vi "Homescreen.vi"() -> ()   [LabVIEW 2015]
uses:
  Home tab state.ctl
  Home state.ctl
  Undelivered instance.ctl
  <vilib>/Utility/sysdir.llb/System Directory Type.ctl
  <vilib>/Utility/config.llb/NI_LVConfig.lvlib
panel:
  out "Tab Control":T1
  in  "Month Cancel":bool
  in  "Month next":bool
  in  "Month reset":bool
  in  "Year":i32=1900
  in  "Month":i32(ring) items=["January", "February", "March", "April", "May", "June", "July", "August", "September", "October", "November", "December"]
  in  "Undelivered instances":i32(listbox)
  out "Total cost":dbl
  in  "Undelivered cancel":bool
  in  "Undelivered Back":bool
  in  "Undelivered next":bool
  in  "Undelivered clear":bool
  in  "Undelivered add":bool
  in  "Undelivered remove":bool
  in  "Save back":bool
  in  "Save exit":bool
  out "Successfully copied":string caption="Config Message"
  in  "Breakdown copy":bool
  out "Breakdown by newspaper":string
  # "This app calculates the total cost of your newspapers for a given month. Please select the month and year you would like to calculate for and then click Next. You will then\nbe able to enter the details of any instances where newspaper(s) were not delivered."
  # "Please enter the details of instances of missing deliveries (if any) and then click Next. You will then be able to copy the break-down and save the data.\n\nClick Add instance to add an instance, and Remove instance to delete the selected instance."
  # "The box below shows you the costs broken down by newspaper. Click Copy to clipboard and save to records to save this to the logs, and copy it to the clipboard.\n\nClick Exit to finish and close the application."
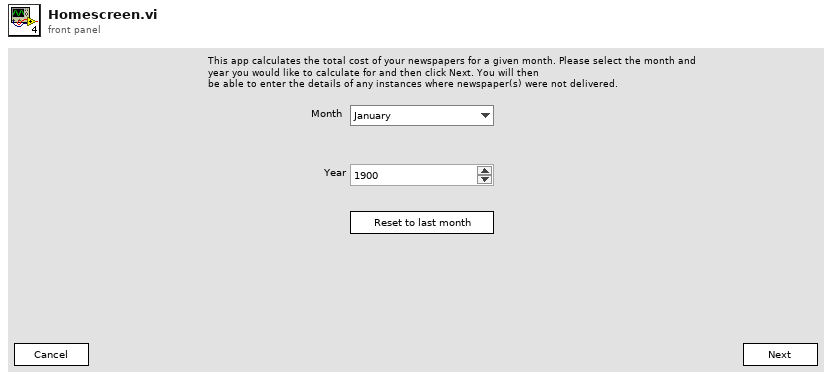
[diagram p1: front panel]
types:
  T1 = typedef "Home tab state.ctl" = enum32{"Pick month", "Select undelivered", "Copy and save"}
  T2 = typedef "Undelivered instance.ctl" = cluster{"Dates":timestamp[], "Newspaper":string}
  T3 = typedef "Home state.ctl" = enum16{"Init", "Open files", "Pick month", "Enter undelivered", "Copy and save", "Exit"}
  T4 = typedef "System Directory Type.ctl" = i32
  T5 = typedef "NI_LVConfig.lvlib/Config Data RefNum.ctl" = refnum<k1>
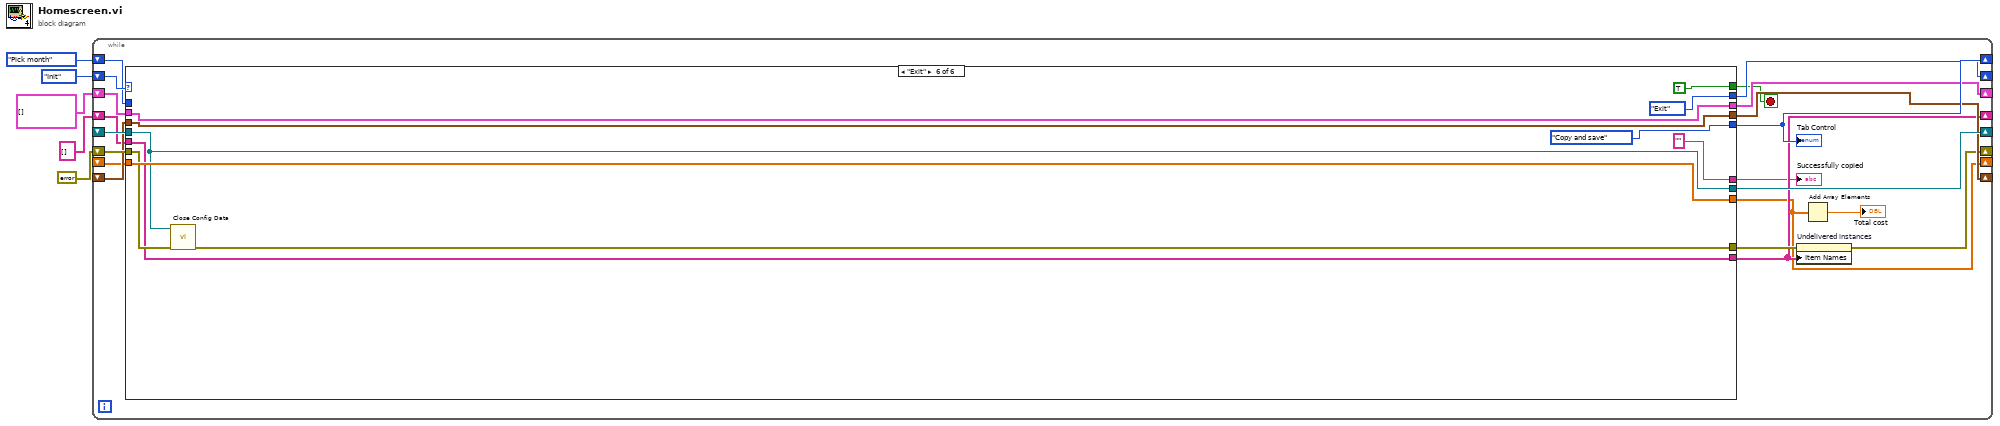
[diagram p0: block diagram]
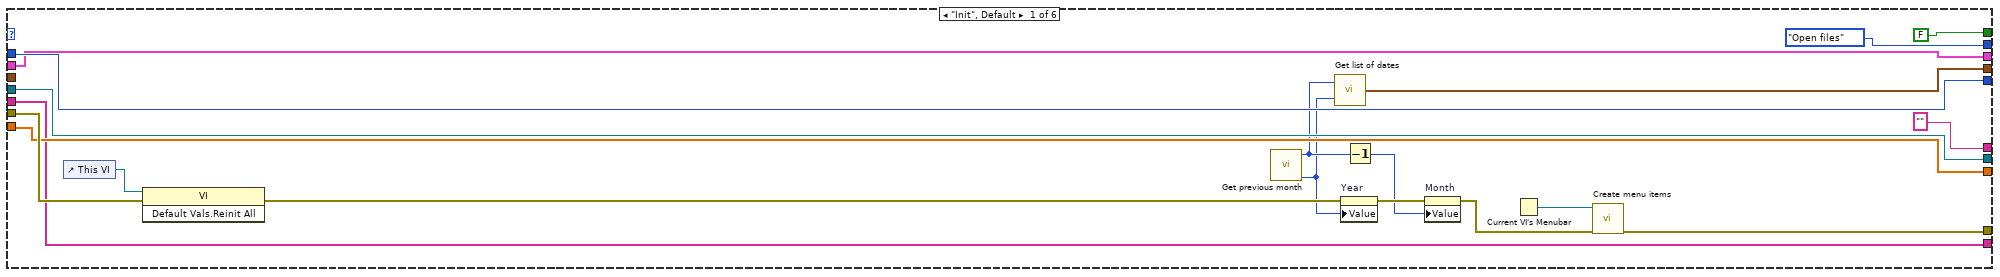
[diagram p2: hidden frame]
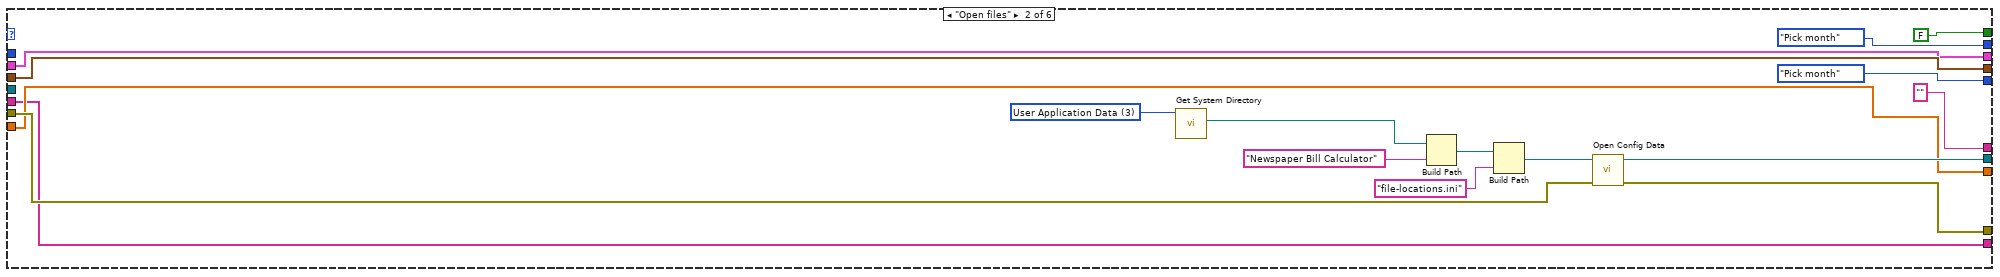
[diagram p3: hidden frame]
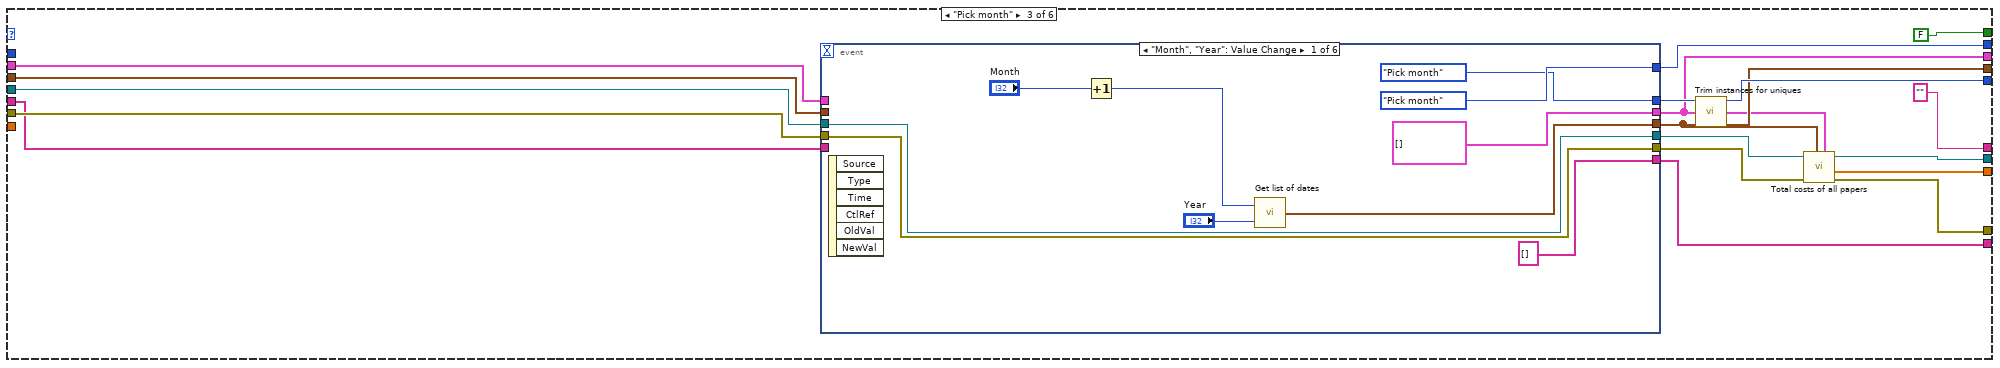
[diagram p4: hidden frame]
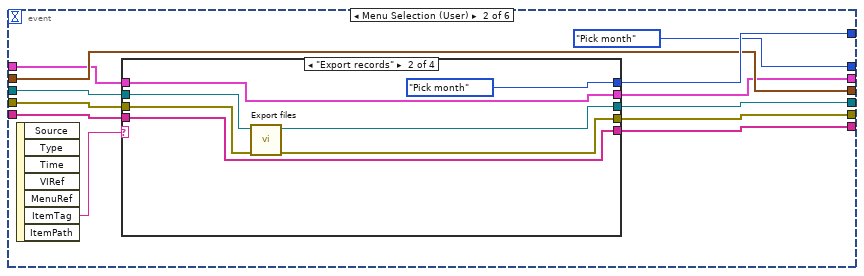
[diagram p5: hidden frame]
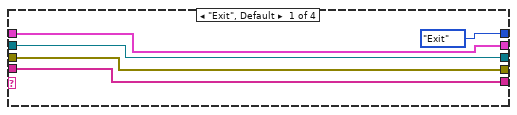
[diagram p6: hidden frame]
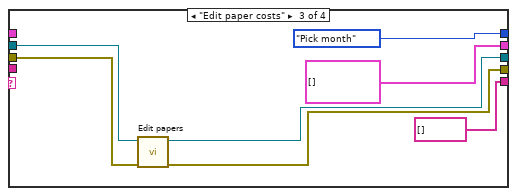
[diagram p7: hidden frame]
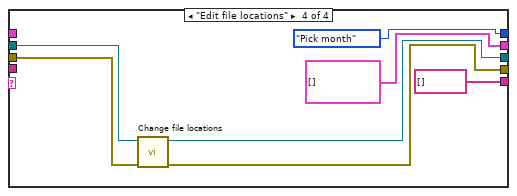
[diagram p8: hidden frame]
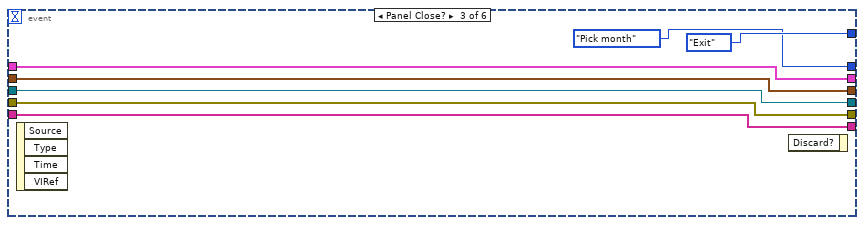
[diagram p9: hidden frame]
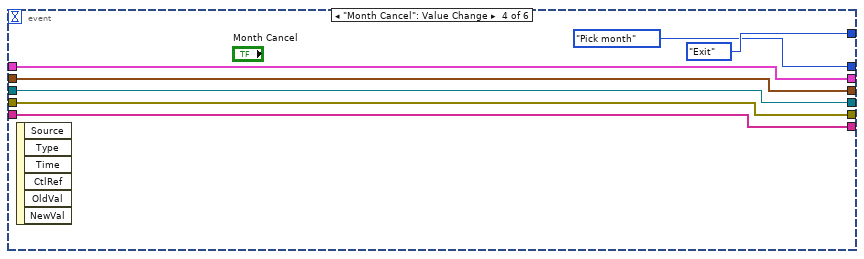
[diagram p10: hidden frame]
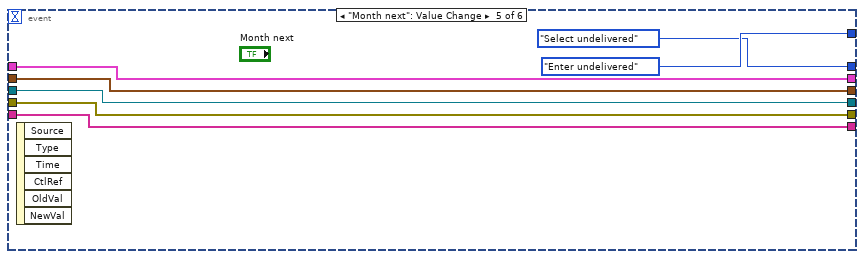
[diagram p11: hidden frame]
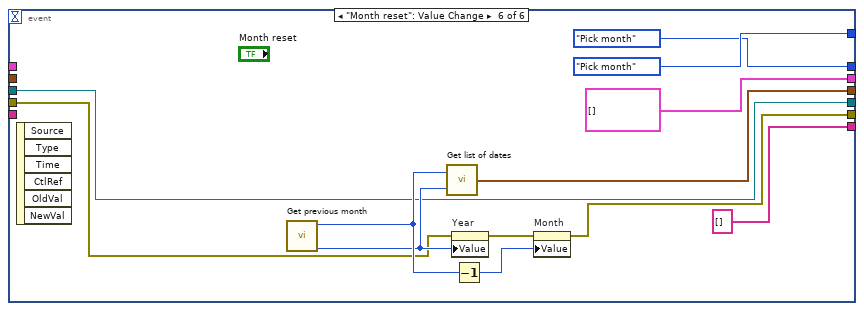
[diagram p12: hidden frame]
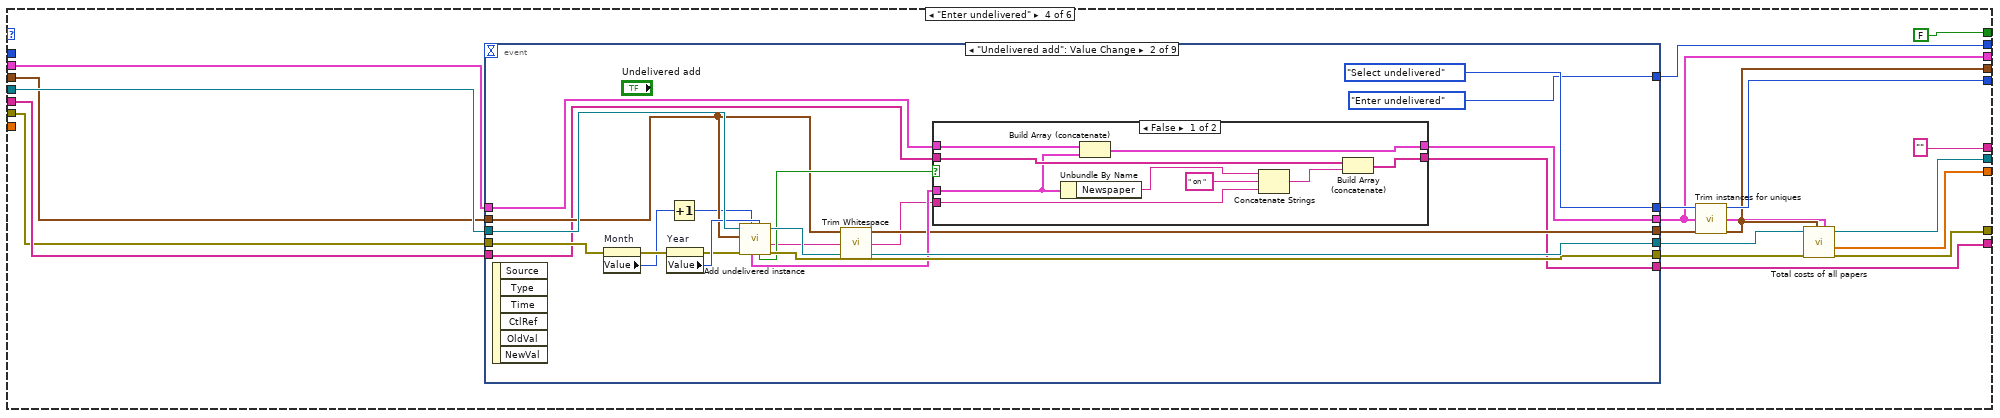
[diagram p13: hidden frame]
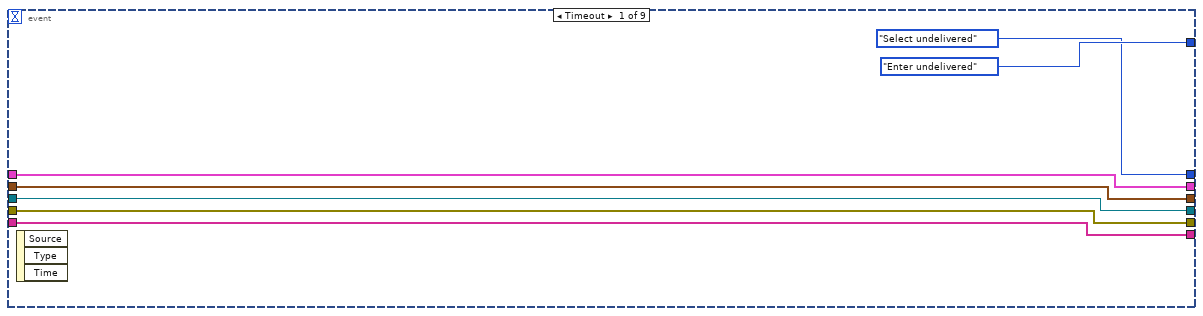
[diagram p14: hidden frame]
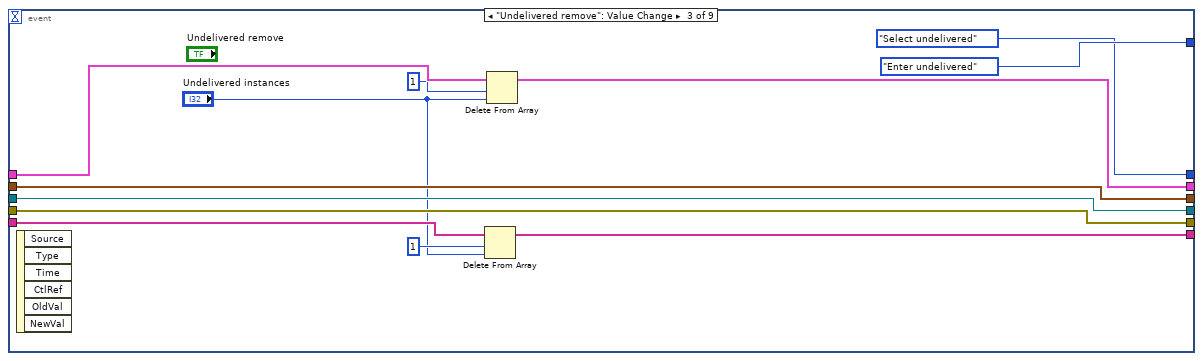
[diagram p16: hidden frame]
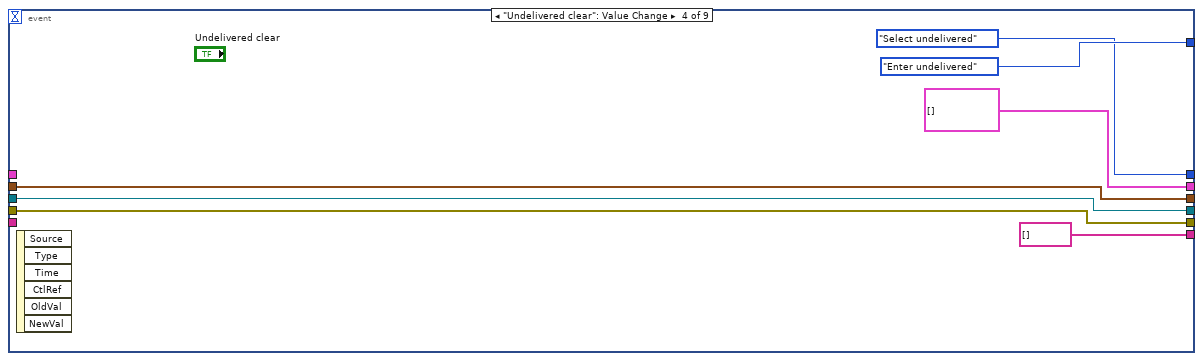
[diagram p17: hidden frame]
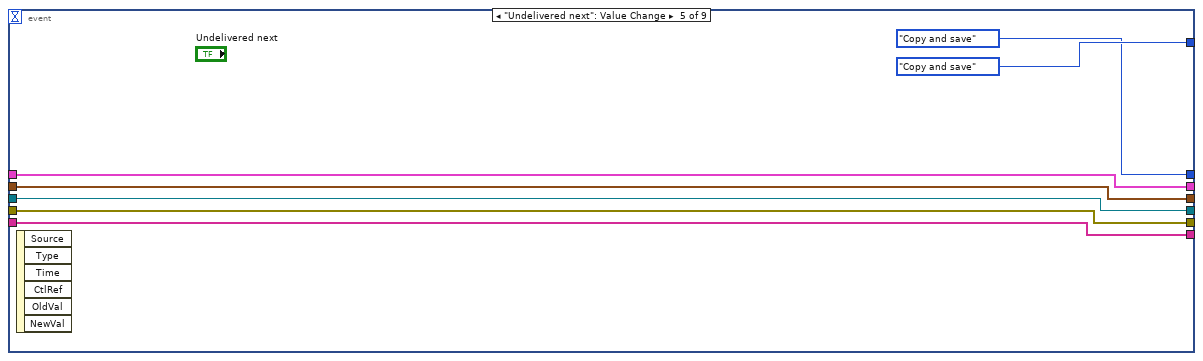
[diagram p18: hidden frame]
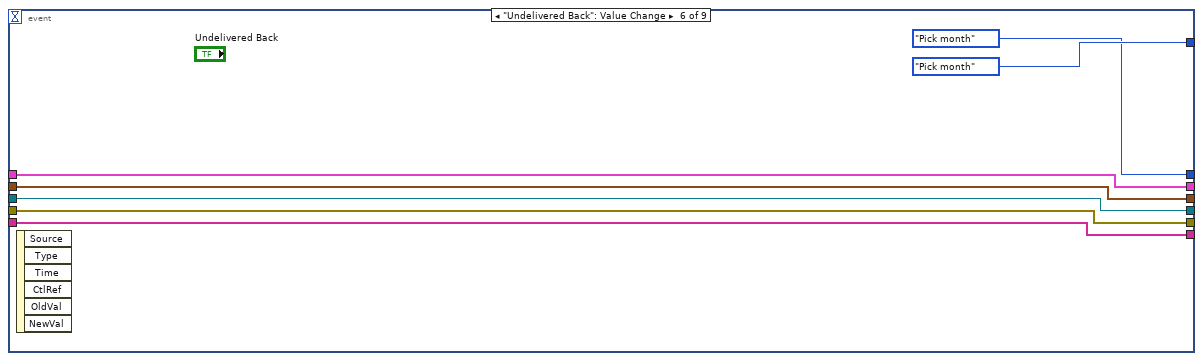
[diagram p19: hidden frame]
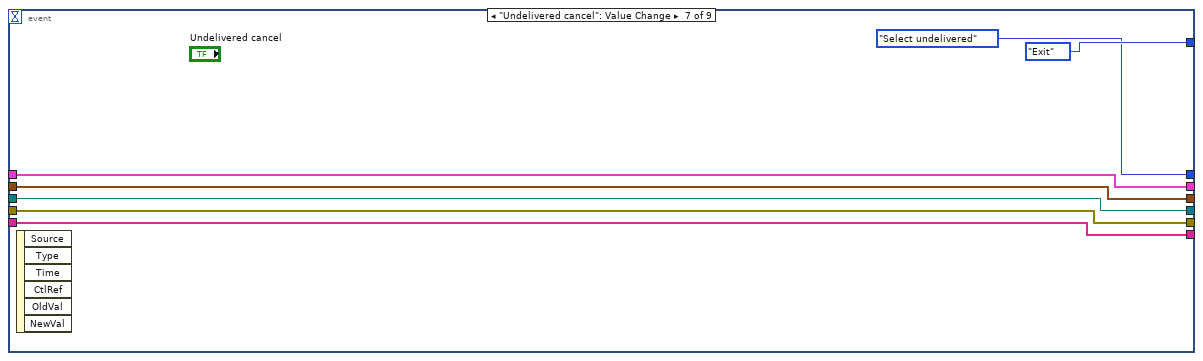
[diagram p20: hidden frame]
diagram:
  n1 = while {
    shift-right: [w22] -> _
    shift-left: Home_state."Init" -> [w25]
    shift-right: [w24] -> _
    shift-left: Home_tab_state."Pick month" ("Tab Control 2") -> [w23]
    shift-right: [w15] -> _
    shift-left: errorcluster {"status"=FALSE, "code"=0, "source"=""} ("error constant") -> [w21]
    shift-right: [w20] -> _
    shift-left: _ -> [w19]
    shift-right: [w18] -> _
    shift-left: _ -> [w17]
    shift-right: [w13] -> _
    shift-left: T2[] [] -> [w14]
    shift-right: [w11] -> _
    shift-left: string[] [] -> [w12]
    shift-right: [w10] -> _
    shift-left: _ -> [w8]
    stop <- w6 stop-if-true
    n2 = case shown="\"Exit\"" w25 {
      tunnel: [w44 Home_tab_state."Pick month" ("Tab Control 2") w70 w173 w305 Home_tab_state."Copy and save" ("Tab Control 2")] -> w24
      tunnel: w23 -> [w44 _ _ _ _ _]
      tunnel: [Home_state."Open files" Home_state."Pick month" w78 w176 w311 Home_state."Exit"] -> w22
      tunnel: w21 -> [w40 w61 w77 w171 w324 w426]
      tunnel: [w36 w54 w64 w163 w315 w424] -> w16
      tunnel: [w34 w53 w63 w162 w313 w425] -> w20
      tunnel: w19 -> [w34 _ w73 w172 w325 w425]
      tunnel: [w26 w49 w69 w168 w307 w427] -> w18
      tunnel: w17 -> [_ w49 w79 w170 w307 w427]
      tunnel: w14 -> [w32 w48 w74 w169 w316 w421]
      tunnel: [w32 w48 w68 w166 w310 w421] -> w13
      tunnel: w12 -> [w30 w50 w75 w178 w308 w422]
      tunnel: [w30 w50 w76 w177 w309 w422] -> w11
      tunnel: [w33 w51 w67 w161 w314 w430] -> w10
      tunnel: w8 -> [w33 w51 _ _ w314 w430]
      tunnel: ["" "" "" "" w317 ""] -> w7
      tunnel: [FALSE FALSE FALSE FALSE FALSE TRUE] -> w6
      frame "Init", Default {
        n3 = control-ref of="This VI"() -> (w38:refnum<vi>)
        n4 = invoke class="VI" method="Default Vals.Reinit All"(reference=w38, error in=w40) -> (error out=w39:errorcluster)  [unwired: 1 in, 2 out]
        n5 = call "Get previous month.vi"() -> ("Year"=w27:i32, "Month (1-12)"=w28:i32)  [unwired: 10 in]
        n6 = call "Get list of dates.vi"("Year"=w27, "Month"=w28) -> ("List"=w26:timestamp[])
        n7 = property on="Year" class="DigNum (strict)"(error in=w39, "Value"=w27) -> (error out=w42:errorcluster)  [unwired: 1 in, 1 out]
        n8 = Decrement(x=w28) -> (x-1=w41:i32)
        n9 = property on="Month" class="Ring (strict)"(error in=w42, "Value"=w41) -> (error out=w37:errorcluster)  [unwired: 1 in, 1 out]
        n10 = Current VI's Menubar() -> (w35:refnum<k9>)
        n11 = call "Create menu items.vi"("Error In"=w37, "Menu ref in"=w35) -> ("Error Out"=w36:errorcluster)  [unwired: 8 in, 1 out]
      }
      frame "Open files" {
        w58 = T4 3 items=["User Home"=0, "User Desktop"=1, "User Documents"=2, "User Application Data"=3, "User Preferences"=4, "User Temporary"=5, "Public Documents"=6, "Public Application Data"=7, "Public Preferences"=8, "Public Cache"=13, "System Core Libraries"=9, "System Installed Libraries"=10, "Application Files"=11, "Boot Volume Root"=12] ("system directory type")
        n12 = call <vilib>:"Get System Directory.vi"("system directory type"=w58) -> ("system directory"=w59:path)  [unwired: 10 in]
        n13 = Build Path(base path=w59, name or relative path="Newspaper Bill Calculator") -> (appended path=w60:path)
        n14 = Build Path(base path=w60, name or relative path="file-locations.ini") -> (appended path=w55:path)
        n15 = call <vilib>:"Open Config Data.vi"("error in (no error)"=w61, "configuration file path"=w55) -> ("error out"=w54:errorcluster, "refnum"=w53:T5)  [unwired: 7 in, 1 out]
      }
      frame "Pick month" {
        n16 = event shown="[0] \"Month\", \"Year\": Value Change" {
          selector: _ -> [_ _ _ _ _ _]
          dyn-events: _ -> [_ _ _ _ _ _]
          timeout: _ -> [_ _ _ _ _ _]
          tunnel: [w89 w95 w132 w141 w147 w153] -> w69
          tunnel: w79 -> [_ w95 w132 w141 w147 _]
          tunnel: [Home_state."Pick month" w96 Home_state."Exit" Home_state."Exit" Home_state."Enter undelivered" Home_state."Pick month"] -> w78
          tunnel: w77 -> [w87 w99 w133 w139 w146 w155]
          tunnel: [w87 w97 w133 w139 w146 w154] -> w65
          tunnel: [T2[] [] w94 w130 w137 w144 T2[] []] -> w68
          tunnel: [string[] [] w92 w131 w138 w145 string[] []] -> w76
          tunnel: w75 -> [_ w91 w131 w138 w145 _]
          tunnel: w74 -> [_ w93 w130 w137 w144 _]
          tunnel: w73 -> [w84 w100 w129 w136 w143 w150]
          tunnel: [w84 w98 w129 w136 w143 w150] -> w66
          tunnel: [Home_tab_state."Pick month" ("Tab Control 2") Home_tab_state."Pick month" ("Tab Control 2") Home_tab_state."Pick month" ("Tab Control 2") Home_tab_state."Pick month" ("Tab Control 2") Home_tab_state."Select undelivered" ("Tab Control 2") Home_tab_state."Pick month" ("Tab Control 2")] -> w70
          event "Month", "Year": Value Change {
            n17 = event-data() -> ()  [unwired: 1 in, 6 out]
            n18 = Increment(x="Month") -> (x+1=w80:i32)
            n19 = call "Get list of dates.vi"("Year"="Year", "Month"=w80) -> ("List"=w89:timestamp[])
          }
          event Menu Selection (User) {
            n20 = event-data() -> ("ItemTag"=w101:string)  [unwired: 1 in, 6 out]
            n21 = case shown="\"Export records\"" w101 {
              tunnel: w100 -> [w104 w113 w120 w126]
              tunnel: w99 -> [w105 w112 w119 w125]
              tunnel: [w104 w111 w117 w123] -> w98
              tunnel: [w105 w110 w118 w124] -> w97
              tunnel: [Home_state."Exit" Home_state."Pick month" Home_state."Pick month" Home_state."Pick month"] -> w96
              tunnel: [w103 w108 T2[] [] T2[] []] -> w94
              tunnel: w93 -> [w103 w108 _ _]
              tunnel: [w102 w107 string[] [] string[] []] -> w92
              tunnel: w91 -> [w102 w107 _ _]
              frame "Exit", Default {
              }
              frame "Export records" {
                n22 = call "Export files.vi"("Error In"=w112, "INI ref in"=w113) -> ("Error Out"=w110:errorcluster, "INI ref out"=w111:T5)  [unwired: 8 in]
              }
              frame "Edit paper costs" {
                n23 = call "Edit papers.vi"("Error In"=w119, "INI refnum in"=w120) -> ("Error Out"=w118:errorcluster, "INI refnum Out"=w117:T5)  [unwired: 8 in]
              }
              frame "Edit file locations" {
                n24 = call "Change file locations.vi"("Error In"=w125, "INI ref in"=w126) -> ("Error Out"=w124:errorcluster, "INI ref out"=w123:T5)  [unwired: 8 in]
              }
            }
          }
          event Panel Close? {
            n25 = event-data() -> ()  [unwired: 1 in, 4 out]
            n26 = event-data() -> ()  [unwired: 2 in, 1 out]
          }
          event "Month Cancel": Value Change {
            n27 = event-data() -> ()  [unwired: 1 in, 6 out]
          }
          event "Month next": Value Change {
            n28 = event-data() -> ()  [unwired: 1 in, 6 out]
          }
          event "Month reset": Value Change {
            n29 = event-data() -> ()  [unwired: 1 in, 6 out]
            n30 = call "Get previous month.vi"() -> ("Year"=w156:i32, "Month (1-12)"=w157:i32)  [unwired: 10 in]
            n31 = call "Get list of dates.vi"("Year"=w156, "Month"=w157) -> ("List"=w153:timestamp[])
            n32 = property on="Year" class="DigNum (strict)"(error in=w155, "Value"=w156) -> (error out=w159:errorcluster)  [unwired: 1 in, 1 out]
            n33 = Decrement(x=w157) -> (x-1=w158:i32)
            n34 = property on="Month" class="Ring (strict)"(error in=w159, "Value"=w158) -> (error out=w154:errorcluster)  [unwired: 1 in, 1 out]
          }
        }
        n35 = call "Trim instances for uniques.vi"("Undelivered instances in"=w68) -> ("Undelivered instances out"=w62:T2[])
        n36 = call "Total costs of all papers.vi"("Instances in"=w62, "Month days in"=w69, "error in (no error)"=w65, "Refnum in"=w66) -> ("error out"=w64:errorcluster, "Total costs"=w67:dbl[], "Refnum out"=w63:T5)  [unwired: 3 in]
      }
      frame "Enter undelivered" {
        n37 = event shown="[1] \"Undelivered add\": Value Change" {
          selector: _ -> [_ _ _ _ _ _ _ _ _]
          dyn-events: _ -> [_ _ _ _ _ _ _ _ _]
          timeout: _ -> [_ _ _ _ _ _ _ _ _]
          tunnel: w172 -> [w184 w205 w220 w231 w238 w246 w253 w260 w273]
          tunnel: w171 -> [w183 w201 w221 w232 w239 w244 w251 w258 w274]
          tunnel: w170 -> [w182 w193 w222 w233 w237 w245 w252 w259 w267]
          tunnel: [w184 w199 w220 w231 w238 w246 w253 w260 w268] -> w165
          tunnel: [w183 w198 w221 w232 w239 w244 w251 w258 w269] -> w164
          tunnel: w169 -> [w185 w197 w227 _ w241 w248 w255 w262 w272]
          tunnel: [w185 w195 w224 T2[] [] w241 w248 w255 w262 w266] -> w166
          tunnel: [w182 w193 w222 w233 w237 w245 w252 w259 w267] -> w168
          tunnel: w178 -> [w180 w192 w228 _ w240 w247 w254 w261 w271]
          tunnel: [w180 w190 w223 string[] [] w240 w247 w254 w261 w270] -> w177
          tunnel: [Home_state."Enter undelivered" Home_state."Enter undelivered" Home_state."Enter undelivered" Home_state."Enter undelivered" Home_state."Copy and save" Home_state."Pick month" Home_state."Exit" Home_state."Exit" w265] -> w176
          tunnel: [Home_tab_state."Select undelivered" ("Tab Control 2") Home_tab_state."Select undelivered" ("Tab Control 2") Home_tab_state."Select undelivered" ("Tab Control 2") Home_tab_state."Select undelivered" ("Tab Control 2") Home_tab_state."Copy and save" ("Tab Control 2") Home_tab_state."Pick month" ("Tab Control 2") Home_tab_state."Select undelivered" ("Tab Control 2") Home_tab_state."Select undelivered" ("Tab Control 2") Home_tab_state."Select undelivered" ("Tab Control 2")] -> w173
          event Timeout {
            n38 = event-data() -> ()  [unwired: 1 in, 3 out]
          }
          event "Undelivered add": Value Change {
            n39 = event-data() -> ()  [unwired: 1 in, 6 out]
            n40 = property on="Month" class="Ring (strict)"(error in=w201) -> (error out=w204:errorcluster, "Value"=w202:i32)  [unwired: 1 in, 1 out]
            n41 = property on="Year" class="DigNum (strict)"(error in=w204) -> (error out=w200:errorcluster, "Value"=w203:i32)  [unwired: 1 in, 1 out]
            n42 = Increment(x=w202) -> (x+1=w187:i32)
            n43 = call "Add undelivered instance.vi"("Year"=w203, "Month"=w187, "Error In"=w200, "Dates in"=w193, "INI Ref in"=w205) -> ("Error Out"=w198:errorcluster, "User"=w191:string, "INI Ref out"=w199:T5, "Cancelled?"=w194:bool, "Paper instance"=w196:T2)  [unwired: 1 in, 1 out]
            n44 = call <vilib>:"Trim Whitespace.vi"("string"=w191) -> ("trimmed string"=w186:string)  [unwired: 1 in]
            n45 = case shown="False" w194 {
              tunnel: w197 -> [w214 w216]
              tunnel: w196 -> [w210 _]
              tunnel: [w213 w216] -> w195
              tunnel: w192 -> [w212 w215]
              tunnel: w186 -> [w207 _]
              tunnel: [w211 w215] -> w190
              frame False {
                n46 = Unbundle By Name(w210) -> ("Newspaper"=w209:string)
                n47 = Build Array (concatenate)(w214, w210) -> (w213:T2[])
                n48 = Concatenate Strings(w209, " on " ("string"), w207) -> (w206:string)
                n49 = Build Array (concatenate)(w212, w206) -> (w211:string[])
              }
              frame True {
              }
            }
          }
          event "Undelivered remove": Value Change {
            n50 = event-data() -> ()  [unwired: 1 in, 6 out]
            n51 = Delete From Array(array=w228, length=1, index="Undelivered instances") -> (array with subset deleted=w223:string[])  [unwired: 1 out]
            n52 = Delete From Array(array=w227, length=1, index="Undelivered instances") -> (array with subset deleted=w224:T2[])  [unwired: 1 out]
          }
          event "Undelivered clear": Value Change {
            n53 = event-data() -> ()  [unwired: 1 in, 6 out]
          }
          event "Undelivered next": Value Change {
            n54 = event-data() -> ()  [unwired: 1 in, 6 out]
          }
          event "Undelivered Back": Value Change {
            n55 = event-data() -> ()  [unwired: 1 in, 6 out]
          }
          event "Undelivered cancel": Value Change {
            n56 = event-data() -> ()  [unwired: 1 in, 6 out]
          }
          event Panel Close? {
            n57 = event-data() -> ()  [unwired: 1 in, 4 out]
            n58 = event-data() -> ()  [unwired: 2 in, 1 out]
          }
          event Menu Selection (User) {
            n59 = event-data() -> ("ItemTag"=w275:string)  [unwired: 1 in, 5 out]
            n60 = case shown="\"Edit paper costs\"" w275 {
              tunnel: w273 -> [w278 w287 w294 w300]
              tunnel: w274 -> [w279 w286 w293 w299]
              tunnel: [w278 w285 w291 w297] -> w268
              tunnel: [w279 w284 w292 w298] -> w269
              tunnel: [Home_state."Exit" Home_state."Enter undelivered" Home_state."Enter undelivered" Home_state."Enter undelivered"] -> w265
              tunnel: [w277 w282 T2[] [] T2[] []] -> w266
              tunnel: w272 -> [w277 w282 _ _]
              tunnel: [w276 w281 string[] [] string[] []] -> w270
              tunnel: w271 -> [w276 w281 _ _]
              frame "Exit", Default {
              }
              frame "Export records" {
                n61 = call "Export files.vi"("Error In"=w286, "INI ref in"=w287) -> ("Error Out"=w284:errorcluster, "INI ref out"=w285:T5)  [unwired: 8 in]
              }
              frame "Edit paper costs" {
                n62 = call "Edit papers.vi"("Error In"=w293, "INI refnum in"=w294) -> ("Error Out"=w292:errorcluster, "INI refnum Out"=w291:T5)  [unwired: 8 in]
              }
              frame "Edit file locations" {
                n63 = call "Change file locations.vi"("Error In"=w299, "INI ref in"=w300) -> ("Error Out"=w298:errorcluster, "INI ref out"=w297:T5)  [unwired: 8 in]
              }
            }
          }
        }
        n64 = call "Trim instances for uniques.vi"("Undelivered instances in"=w166) -> ("Undelivered instances out"=w167:T2[])
        n65 = call "Total costs of all papers.vi"("Instances in"=w167, "Month days in"=w168, "error in (no error)"=w164, "Refnum in"=w165) -> ("error out"=w163:errorcluster, "Total costs"=w161:dbl[], "Refnum out"=w162:T5)  [unwired: 3 in]
      }
      frame "Copy and save" {
        n66 = call "Read paper data.vi"("Refnum in"=w325, "error in (no error)"=w324) -> ("Names"=w323:string[], "Refnum out"=w312:T5, "error out"=w319:errorcluster)  [unwired: 9 in, 2 out]
        n67 = for {
          tunnel: w323 -> [w419] mode=indexing
          tunnel: w314 -> [w414] mode=indexing
          shift-right: [w415] -> w321
          shift-left: "" -> [w416]
          n68 = Format Into String(format string="%#f", w414) -> (resulting string=w413:string)  [unwired: 2 in, 1 out]
          n69 = Concatenate Strings(w416, w419, ": " ("string"), w413, "\n") -> (w415:string)
        }
        n70 = Add Array Elements(numeric array=w314) -> (sum=w304:dbl)
        n71 = Format Into String(format string="%#f", w304) -> (resulting string=w303:string)  [unwired: 2 in, 1 out]
        n72 = Concatenate Strings(w321, "TOTAL: " ("string"), w303) -> (w318:string)
        "Breakdown by newspaper" <- w318
        n73 = event shown="[1] \"Breakdown copy\": Value Change" {
          selector: _ -> [_ _ _ _ _ _]
          dyn-events: _ -> [_ _ _ _ _ _]
          timeout: _ -> [_ _ _ _ _ _]
          tunnel: w319 -> [w330 w351 w356 w363 w370 w380]
          tunnel: w318 -> [_ w350 _ _ _ w381]
          tunnel: ["" "Successfully copied and saved!" "" "" "" ""] -> w317
          tunnel: w316 -> [w327 w335 w353 w361 w367 w382]
          tunnel: [w330 w340 w356 w363 w370 w377] -> w315
          tunnel: w314 -> [_ w342 _ _ _ _]
          tunnel: [w331 w339 w357 w364 w371 w378] -> w313
          tunnel: w312 -> [w331 w338 w357 w364 w371 w379]
          tunnel: [Home_state."Copy and save" ("Enum") Home_state."Copy and save" ("Enum") Home_state."Enter undelivered" ("Enum") Home_state."Exit" ("Enum") Home_state."Exit" ("Enum") w384] -> w311
          tunnel: [w327 w335 w353 w361 w367 w383] -> w310
          tunnel: [w328 w336 w354 w360 w368 w376] -> w309
          tunnel: w308 -> [w328 w336 w354 w360 w368 w374]
          tunnel: [Home_tab_state."Copy and save" ("Tab Control 2") Home_tab_state."Copy and save" ("Tab Control 2") Home_tab_state."Select undelivered" ("Tab Control 2") Home_tab_state."Copy and save" ("Tab Control 2") Home_tab_state."Copy and save" ("Tab Control 2") Home_tab_state."Copy and save" ("Tab Control 2")] -> w305
          event Timeout {
            n74 = event-data() -> ()  [unwired: 1 in, 3 out]
          }
          event "Breakdown copy": Value Change {
            n75 = event-data() -> ()  [unwired: 1 in, 6 out]
            n76 = invoke class="App" method="Clipboard.Write"(error in=w351, "Param 0"=w350) -> (error out=w348:errorcluster)  [unwired: 2 in, 3 out]
            n77 = property on="Month" class="Ring (strict)"(error in=w348) -> (error out=w345:errorcluster, "Value"=w344:i32)  [unwired: 1 in, 1 out]
            n78 = property on="Year" class="DigNum (strict)"(error in=w345) -> (error out=w341:errorcluster, "Value"=w343:i32)  [unwired: 1 in, 1 out]
            n79 = Increment(x=w344) -> (x+1=w333:i32)
            n80 = call "Write record log.vi"("Year"=w343, "Month"=w333, "Instances in"=w335, "Error In"=w341, "refnum"=w338) -> ("Error Out"=w347:errorcluster, "refnum out"=w346:T5)  [unwired: 5 in]
            n81 = call "Write cost log.vi"("Year"=w343, "Month"=w333, "Costs in"=w342, "error in (no error)"=w347, "Refnum in"=w346) -> ("error out"=w340:errorcluster, "Refnum out"=w339:T5)  [unwired: 5 in]
          }
          event "Save back": Value Change {
            n82 = event-data() -> ()  [unwired: 1 in, 6 out]
          }
          event "Save exit": Value Change {
            n83 = event-data() -> ()  [unwired: 1 in, 6 out]
          }
          event Panel Close? {
            n84 = event-data() -> ()  [unwired: 1 in, 4 out]
            n85 = event-data() -> ()  [unwired: 2 in, 1 out]
          }
          event Menu Selection? (App) {
            n86 = event-data() -> ("ItemTag"=w385:string)  [unwired: 1 in, 5 out]
            n87 = case shown="\"Exit\", Default" w385 {
              tunnel: w379 -> [w388 w397 w404 w410]
              tunnel: w380 -> [w389 w396 w403 w409]
              tunnel: [w388 w395 w401 w407] -> w378
              tunnel: [w389 w394 w402 w408] -> w377
              tunnel: [Home_state."Exit" Home_state."Copy and save" Home_state."Copy and save" Home_state."Copy and save"] -> w384
              tunnel: [w387 w392 T2[] [] T2[] []] -> w383
              tunnel: w382 -> [w387 w392 _ _]
              tunnel: w381 -> [_ _ _ _]
              tunnel: [w386 w391 string[] [] string[] []] -> w376
              tunnel: w374 -> [w386 w391 _ _]
              frame "Exit", Default {
              }
              frame "Export records" {
                n88 = call "Export files.vi"("Error In"=w396, "INI ref in"=w397) -> ("Error Out"=w394:errorcluster, "INI ref out"=w395:T5)  [unwired: 8 in]
              }
              frame "Edit paper costs" {
                n89 = call "Edit papers.vi"("Error In"=w403, "INI refnum in"=w404) -> ("Error Out"=w402:errorcluster, "INI refnum Out"=w401:T5)  [unwired: 8 in]
              }
              frame "Edit file locations" {
                n90 = call "Change file locations.vi"("Error In"=w409, "INI ref in"=w410) -> ("Error Out"=w408:errorcluster, "INI ref out"=w407:T5)  [unwired: 8 in]
              }
            }
            n91 = event-data() -> ()  [unwired: 2 in, 1 out]
          }
        }
      }
      frame "Exit" {
        n92 = call <vilib>:"Close Config Data.vi"("error in (no error)"=w426, "refnum"=w425) -> ("error out"=w424:errorcluster)  [unwired: 8 in, 1 out]
      }
    }
    "Tab Control" <- w24
    "Successfully copied" <- w7
    n93 = property on="Undelivered instances" class="LstBox (strict)"(error in=w16, "Item Names"=w11) -> (error out=w15:errorcluster)  [unwired: 1 in, 1 out]
    n94 = Add Array Elements(numeric array=w10) -> (sum=→"Total cost":dbl)
  }
